vi "Lockin_Example_Lockin.vi"() -> ()   [LabVIEW 2016]
uses:
  Typedefs/AO-cluster.ctl
  Typedefs/AO_Amp-array.ctl
  Typedefs/AO_DC-array.ctl
  Typedefs/AO_f-array.ctl
  Typedefs/AO_phi-array.ctl
  Typedefs/Function-array.ctl
  Typedefs/Function-enum.ctl
  Typedefs/REF-cluster.ctl
  Typedefs/REF_f-array.ctl
  Typedefs/REF_phi-array.ctl
panel:
  in  "Channels: Lockin":T1={"REF f (Hz)"=[13.0], "REF phi (deg)"=[0.0]} {"REF phi (deg)" format="%#_3g"}
  out "Lockin vs time":cluster{timestamp[], dbl[]}(graph)
  out "Lockin vs parameter":cluster{"Y":dbl[], "Y":dbl[]}(graph)
  in  "step":dbl=0.025
  in  "end":dbl=0.1
  in  "start":dbl
  in  "Channels: AO":T4={"AO amp (V)"=[0.1, 0.2, 0.0, 0.0, 0.0, 0.0, 0.0, 0.0], "AO DC (V)"=[0.0, 0.0, 0.0, 0.0, 0.0, 0.0, 0.0, 0.0], "AO f (Hz)"=[13.0, 13.0, 13.0, 13.0, 13.0, 13.0, 13.0, 13.0], "AO phi (deg)"=[0.0, 0.0, 0.0, 0.0, 0.0, 0.0, 0.0, 0.0], "function"=[enum."Sine Wave", enum."Sine Wave", enum."Sine Wave", enum."Sine Wave", enum."Sine Wave", enum."Sine Wave", enum."Sine Wave", enum."Sine Wave"]} {"AO f (Hz)" min=0.001 max=10000.0; "AO DC (V)" format="%#_6p"; "AO amp (V)" format="%#_6p"}
  # "Lockin Example: Lockin\nMake Sure Lockin Program is running!"
  # "0"
  # "1"
  # "2"
  # "3"
  # "4"
  # "5"
  # "6"
  # "7"
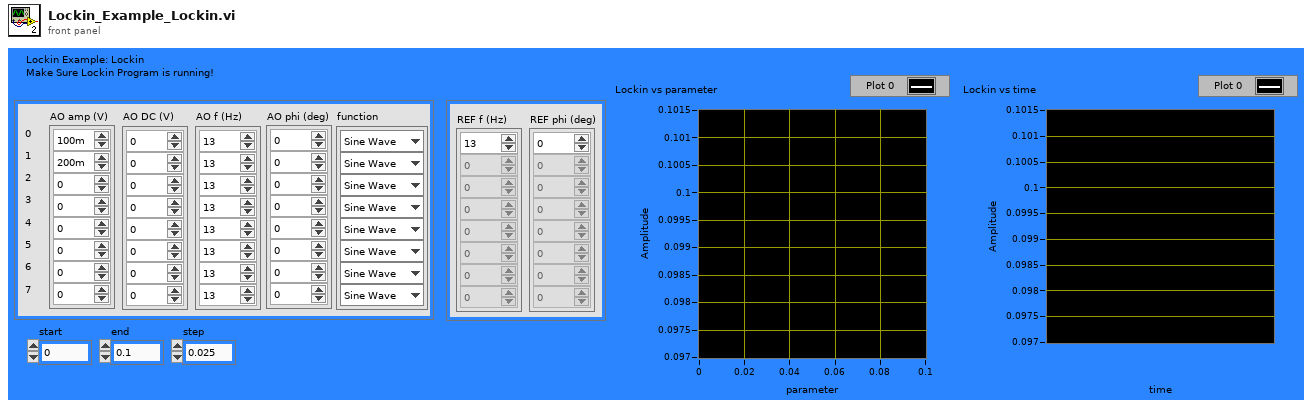
[diagram p1: front panel]
types:
  T1 = typedef "REF-cluster.ctl" = cluster{"REF f (Hz)":T2, "REF phi (deg)":T3}
  T2 = typedef "REF_f-array.ctl" = dbl[]
  T3 = typedef "REF_phi-array.ctl" = dbl[]
  T4 = typedef "AO-cluster.ctl" = cluster{"AO amp (V)":T5, "AO DC (V)":T6, "AO f (Hz)":T7, "AO phi (deg)":T8, "function":T9}
  T5 = typedef "AO_Amp-array.ctl" = dbl[]
  T6 = typedef "AO_DC-array.ctl" = dbl[]
  T7 = typedef "AO_f-array.ctl" = dbl[]
  T8 = typedef "AO_phi-array.ctl" = dbl[]
  T9 = typedef "Function-array.ctl" = T10[]
  T10 = typedef "Function-enum.ctl" = enum16{"Sine Wave", "Triangle Wave", "Square Wave", "Sawtooth Wave"}
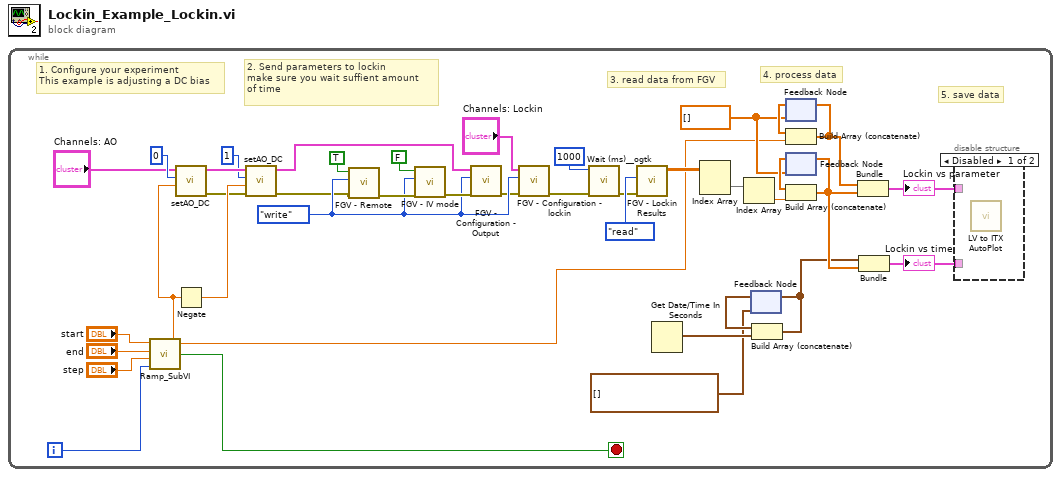
[diagram p0: block diagram]
diagram:
  n1 = while {
    i -> [w36]
    stop <- w39 stop-if-true
    w12 = dbl[] []
    w14 = enum16{"write", "read"}."write" ("Function")
    # "5. save data"
    # "4. process data"
    # "3. read data from FGV"
    # "1. Configure your experiment\nThis example is adjusting a DC bias"
    # "2. Send parameters to lockin\nmake sure you wait suffient amount\nof time"
    n2 = call <userlib>:"Ramp_SubVI.vi"("index"=w36, "step"="step", "end"="end", "start"="start") -> ("Stop?"=w39:bool, "Numeric"=w7:dbl)  [unwired: 1 in]
    n3 = call "setAO_DC.vi"("new DC (V)"=w7, "AO Channel"=0, "Channels: AO"="Channels: AO") -> ("error out"=w4:errorcluster, "Channels: AO"=w10:T4)  [unwired: 7 in]
    n4 = Negate(x=w7) -> (-x=w6:dbl)
    n5 = call "setAO_DC.vi"("error in (no error)"=w4, "new DC (V)"=w6, "AO Channel"=1, "Channels: AO"=w10) -> ("error out"=w3:errorcluster, "Channels: AO"=w2:T4)  [unwired: 6 in]
    n6 = call "FGV - Remote.vi"("error in"=w3, "Function"=w14, "Remote Mode"=TRUE ("IV mode")) -> ("error out"=w18:errorcluster)  [unwired: 3 in, 1 out]
    n7 = call "FGV - IV mode.vi"("error in"=w18, "Function"=w14, "IV mode"=FALSE) -> ("error out"=w19:errorcluster)  [unwired: 3 in, 1 out]
    n8 = call "FGV - Configuration - Output.vi"("error in"=w19, "Function"=w14, "Channels: AO"=w2) -> ("error out"=w13:errorcluster)  [unwired: 3 in, 1 out]
    n9 = call "FGV - Configuration - lockin.vi"("error in"=w13, "Function"=w14, "Channels: Lockin"="Channels: Lockin") -> ("error out"=w15:errorcluster)  [unwired: 3 in, 1 out]
    n10 = call <userlib>:"Wait (ms)__ogtk.vi"("error in (no error)"=w15, "milliseconds to wait"=u32 1000) -> ("error out"=w21:errorcluster)  [unwired: 8 in, 1 out]
    n11 = call "FGV - Lockin Results.vi"("error in"=w21, "Function"=enum16{"write", "read"}."read") -> ("Input Signals"=w31:dbl[][])  [unwired: 4 in, 1 out]
    n12 = Get Date/Time In Seconds() -> (seconds since 1Jan1904=w24:timestamp)
    n13 = Index Array(array=w31) -> (element=w30:dbl[])  [unwired: 2 in]
    n14 = Index Array(array=w30) -> (element=w29:dbl)  [unwired: 1 in]
    n15 = feedback #1(timestamp[] []) -> (w22:timestamp[])
    n16 = Build Array (concatenate)(w22, w24) -> (w23:timestamp[])
    n17 = feedback-in #1(w23) -> ()
    n18 = feedback #2(w12) -> (w26:dbl[])
    n19 = Build Array (concatenate)(w26, w7) -> (w25:dbl[])
    n20 = feedback-in #2(w25) -> ()
    n21 = feedback #3(w12) -> (w28:dbl[])
    n22 = Build Array (concatenate)(w28, w29) -> (w27:dbl[])
    n23 = feedback-in #3(w27) -> ()
    n24 = Bundle(w25, w27) -> (w34:cluster{dbl[], dbl[]})  [unwired: 1 in]
    "Lockin vs parameter" <- w34
    n25 = Bundle(w23, w27) -> (w33:cluster{timestamp[], dbl[]})  [unwired: 1 in]
    "Lockin vs time" <- w33
    n26 = disable-structure shown="Disabled" {
      disable-tunnel: w34 -> [_ _]
      disable-tunnel: w33 -> [_ _]
      frame Disabled {
        n27 = call <userlib>:"LV to ITX AutoPlot.vi"() -> ()  [unwired: 15 in, 1 out]
      }
      frame Enabled {
      }
    }
  }
